vi "main.vi"() -> ()   [LabVIEW 2023]
panel:
  in  "URL":string
  out "output":string
  in  "Numeric":dbl
  out "body":string
  out "headers":string
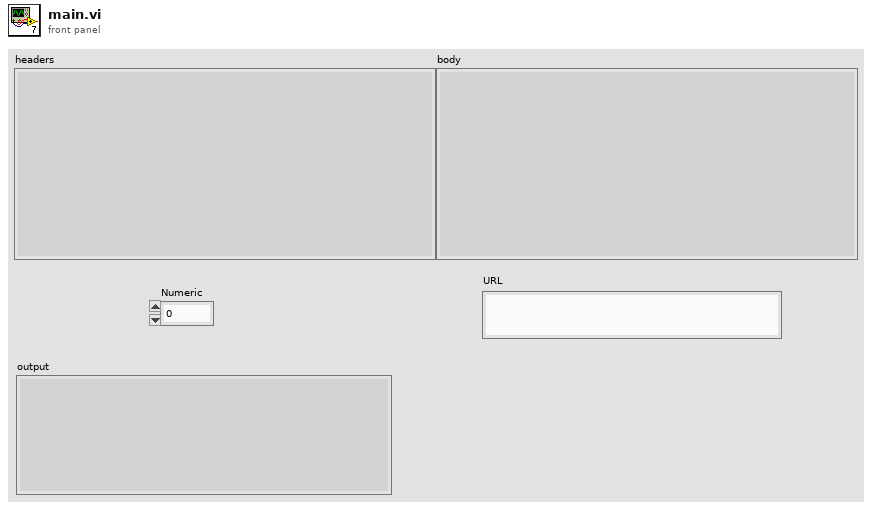
[diagram p1: front panel]
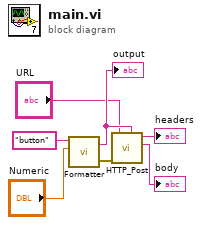
[diagram p0: block diagram]
diagram:
  n1 = call "Formatter.vi"("Variant"="Numeric", "ID"="button" ("string")) -> ("error out"=w3:errorcluster, "output"=w2:string)  [unwired: 2 in]
  "output" <- w2
  n2 = call "HTTP_Post.vi"("data"=w2, "URL"="URL", "error in (no error)"=w3) -> ("body"=→"body":string, "headers"=→"headers":string)  [unwired: 4 in, 1 out]
